vi "Get Name.vi"(8 "error in (no error)":errorcluster, 11 "Forward Drive Cmd in":refnum<class "Forward Drive Cmd.lvclass">) -> (0 "error out":errorcluster, 2 "Command Name":string, 3 "Forward Drive Cmd out":refnum<class "Forward Drive Cmd.lvclass">)   [LabVIEW 2014, in "Forward Drive.lvlib" / "Forward Drive Cmd.lvclass"]
uses:
  Forward Drive Cmd.lvclass
  Robot Actor Framework/Command Actor/Command Actor Class/Command Actor.lvclass
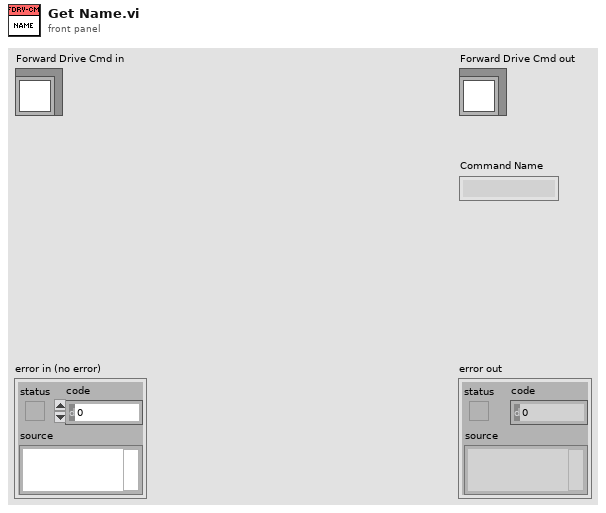
[diagram p1: front panel]
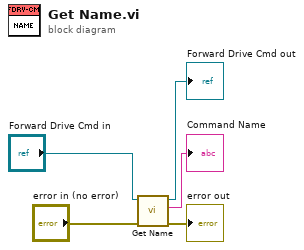
[diagram p0: block diagram]
diagram:
  n1 = call-parent "Get Name.vi"("error in (no error)"="error in (no error)", "Command Actor in"="Forward Drive Cmd in") -> ("error out"=→"error out":errorcluster, "Command Name"=→"Command Name":string, "Command Actor out"=→"Forward Drive Cmd out":refnum<class "Forward Drive Cmd.lvclass">)  [unwired: 7 in]
